vi "Get VI.vi"(8 "error in (no error)":errorcluster, 10 "VI Path (Relative)":string, 11 "ProjectData in":refnum<class "Project Data.lvclass">) -> (0 "error out":errorcluster, 1 "VI Data out":refnum<class "VI Data.lvclass">, 2 "found":bool, 3 "ProjectData out":refnum<class "Project Data.lvclass">)   [LabVIEW 2013, in "SET Project Data.lvlib" / "Project Data.lvclass"]
uses:
  Project Data.lvclass
  VI Class/VI Data.lvclass
  Project Data.lvclass/Project Data.ctl
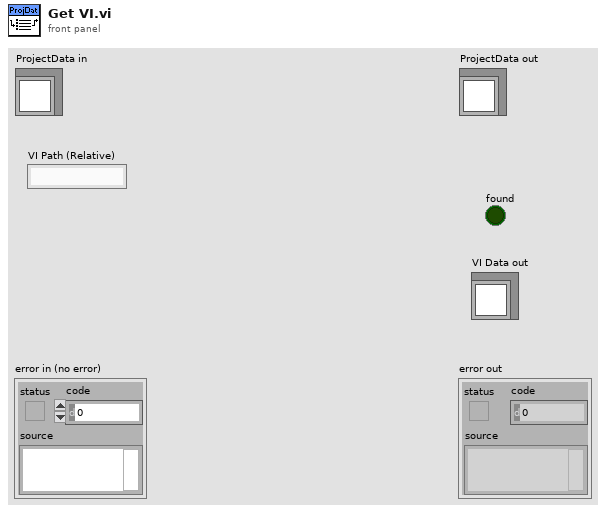
[diagram p1: front panel]
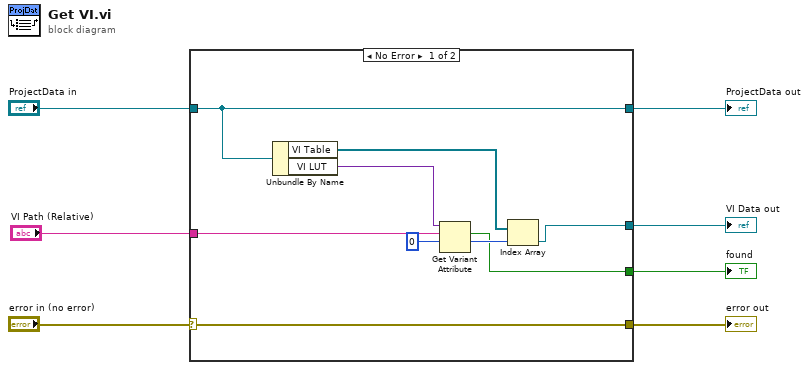
[diagram p0: block diagram]
diagram:
  n1 = case shown="No Error" "error in (no error)" {
    selector: "error in (no error)" -> [w16 w18]
    tunnel: [w16 w18] -> w6
    tunnel: [w11 w17] -> w4
    tunnel: "ProjectData in" -> [w11 w17]
    tunnel: "VI Path (Relative)" -> [w10 _]
    tunnel: [w9 _] -> w2
    tunnel: [w8 _] -> w1
    frame No Error {
      n2 = Unbundle By Name(w11) -> ("VI Table"=w13:refnum<class "VI Data.lvclass">[], "VI LUT"=w15:variant)
      n3 = Get Variant Attribute(Variant=w15, name=w10, default value (empty Variant)=0) -> (found=w9:bool, value=w12:i32)  [unwired: 1 in, 2 out]
      n4 = Index Array(array=w13, index=w12) -> (element=w8:refnum<class "VI Data.lvclass">)
    }
    frame Error {
    }
  }
  "error out" <- w6
  "ProjectData out" <- w4
  "found" <- w2
  "VI Data out" <- w1
